vi "GetParamValue.vi"(2 "Params":T1(array[cluster]), 3 "command":string) -> (0 "default":string, 1 "value":string)   [LabVIEW 2012]
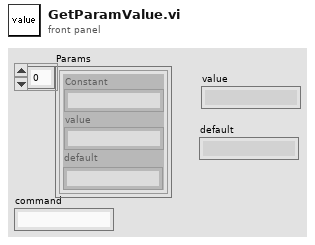
[diagram p1: front panel]
types:
  T1 = cluster{"Constant":string, "value":string, "default":string}[]
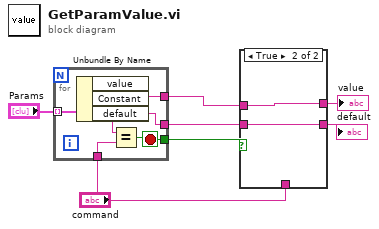
[diagram p0: block diagram]
diagram:
  n1 = for {
    tunnel: "Params" -> [w13] mode=indexing
    tunnel: "command" -> [w11]
    tunnel: [w10] -> w4
    tunnel: [w9] -> w6
    tunnel: [w8] -> w2
    stop <- w9 stop-if-true
    n2 = Unbundle By Name(w13) -> ("value"=w10:string, "Constant"=w12:string, "default"=w8:string)
    n3 = Equal?(x=w12, y=w11) -> (x = y?=w9:bool)
  }
  n4 = case shown="True" w6 {
    tunnel: [w15 w17] -> w5
    tunnel: w4 -> [_ w17]
    tunnel: "command" -> [w15 _]
    tunnel: w2 -> [w14 w16]
    tunnel: [w14 w16] -> w1
    frame False {
    }
    frame True {
    }
  }
  "value" <- w5
  "default" <- w1
